vi "UHR-Fleezers Control (host) - Lorentz v2.vi"() -> ()   [LabVIEW 2014] (continued)
                n3918 = String Subset(string=w6021, length (rest)=w6018) -> (substring=w6017:string)  [unwired: 1 out]
                n3919 = Concatenate Strings(w6017, "_log.txt" ("string")) -> (w6015:string)
                n3920 = String To Path(string=w6015) -> (path=w6011:path)
                n3921 = Open/Create/Replace File(file path (use dialog)=w6011, operation (0:open)=T40."create", access (0:read/write)=enum16{"read/write", "read-only", "write-only"}."write-only") -> (refnum out=w6012:refnum<file>)  [unwired: 1 in, 4 out]
                n3922 = Deny Access(7:w6012) -> (3:w6009:refnum<file>)  [unwired: 1 in, 2 out]
                n3923 = call "write to event log.vi"("log file ref"=w6009, "time"=0.0, "input string"="start log") -> ()  [unwired: 8 in]
              }
            }
            "log file ref" <- w5943
            n3924 = Array Size(array=w5979) -> (size(s)=w5980:i32)
            n3925 = Open/Create/Replace File(file path (use dialog)=w5945, operation (0:open)=T40."create", access (0:read/write)=enum16{"read/write", "read-only", "write-only"}."write-only") -> (refnum out=w5993:refnum<file>)  [unwired: 1 in, 4 out]
            n3926 = local write "Saving..."(TRUE ("Saving...")) -> ()
            n3927 = To Double Precision Float(number=w5980) -> (double precision float=w5978:dbl)
            n3928 = String Length(string="Comment (data description)") -> (length=w5977:i32)
            n3929 = To Double Precision Float(number=w5977) -> (double precision float=w5976:dbl)
            n3930 = Deny Access(7:w5993) -> (3:w5992:refnum<file>)  [unwired: 1 in, 2 out]
            n3931 = Build Array (concatenate)(w5978, w5979, w5976) -> (w5955:dbl[])
            n3932 = case "If fluorescence data to be saved" shown="True" w5968 {
              tunnel: w5945 -> [_ w6074]
              tunnel: [w6044 w6057] -> w5969
              tunnel: [w6044 w6045] -> w5941
              frame False {
                w6044 = refnum<k0> refnum
              }
              frame True {
                w6056 = 0.0
                w6049 = T40."create" ("operation (0:open)")
                w6050 = enum16{"read/write", "read-only", "write-only"}."write-only" ("access (0:read/write)")
                n3933 = local read "APD Integration Time (s)"() -> (w6062:dbl)
                n3934 = local read "N APD Samp/step"() -> (w6055:dbl)
                n3935 = local read "Number of APDs"() -> (w6054:u8)
                n3936 = Path To String(path=w6074) -> (string=w6073:string)
                n3937 = String Length(string=w6073) -> (length=w6072:i32)
                n3938 = Subtract(x=w6072, y=4) -> (x-y=w6070:i32)
                n3939 = String Subset(string=w6073, length (rest)=w6070) -> (substring=w6053:string)  [unwired: 1 out]
                n3940 = Build Array(w6062, w6055, w6054, w6056, w6056, w6056, w6056, w6056) -> (w6059:dbl[])
                n3941 = Concatenate Strings(w6053, "_green.dat") -> (w6051:string)
                n3942 = Concatenate Strings(w6053, "_fl.dat" ("string")) -> (w6068:string)
                n3943 = Array Size(array=w6059) -> (size(s)=w6061:i32)
                n3944 = String To Path(string=w6068) -> (path=w6066:path)
                n3945 = Open/Create/Replace File(file path (use dialog)=w6066, operation (0:open)=w6049, access (0:read/write)=w6050) -> (refnum out=w6067:refnum<file>)  [unwired: 1 in, 4 out]
                n3946 = Deny Access(7:w6067) -> (3:w6063:refnum<file>)  [unwired: 1 in, 2 out]
                n3947 = String To Path(string=w6051) -> (path=w6048:path)
                n3948 = To Double Precision Float(number=w6061) -> (double precision float=w6060:dbl)
                n3949 = Build Array (concatenate)(w6060, w6059) -> (w6058:dbl[])
                n3950 = Write to Binary File(file (use dialog)=w6063, data=w6058, 5:FALSE ("prepend array or string size? (T)"), 9:T41."big-endian, network order" ("byte order (0:big-endian, network order)")) -> (refnum out=w6057:refnum<file>)  [unwired: 1 in, 3 out]
                n3951 = Open/Create/Replace File(file path (use dialog)=w6048, operation (0:open)=w6049, access (0:read/write)=w6050) -> (refnum out=w6046:refnum<file>, error out=w6047:errorcluster)  [unwired: 3 in, 1 out]
                n3952 = Deny Access(4:w6047, 7:w6046) -> (3:w6045:refnum<file>)  [unwired: 1 in, 1 out]
              }
            }
            n3953 = case shown="True" w5957 {
              tunnel: w5945 -> [_ w6029]
              tunnel: [refnum<k0> refnum w6028] -> w5958
              frame False {
              }
              frame True {
                w6024 = 0.0 ("element")
                n3954 = Path To String(path=w6029) -> (string=w6043:string)
                n3955 = Build Array(w6024, w6024, w6024, w6024, w6024, w6024, w6024, w6024) -> (w6025:dbl[])
                n3956 = String Length(string=w6043) -> (length=w6042:i32)
                n3957 = Subtract(x=w6042, y=4) -> (x-y=w6040:i32)
                n3958 = Array Size(array=w6025) -> (size(s)=w6027:i32)
                n3959 = String Subset(string=w6043, length (rest)=w6040) -> (substring=w6039:string)  [unwired: 1 out]
                n3960 = To Double Precision Float(number=w6027) -> (double precision float=w6026:dbl)
                n3961 = Concatenate Strings(w6039, "_pos.dat" ("string")) -> (w6037:string)
                n3962 = Build Array (concatenate)(w6026, w6025) -> (w6023:dbl[])
                n3963 = String To Path(string=w6037) -> (path=w6033:path)
                n3964 = Open/Create/Replace File(file path (use dialog)=w6033, operation (0:open)=T40."create", access (0:read/write)=enum16{"read/write", "read-only", "write-only"}."write-only") -> (refnum out=w6034:refnum<file>)  [unwired: 1 in, 4 out]
                n3965 = Deny Access(7:w6034) -> (3:w6030:refnum<file>)  [unwired: 1 in, 2 out]
                n3966 = Write to Binary File(file (use dialog)=w6030, data=w6023, 5:FALSE ("prepend array or string size? (T)"), 9:T41."big-endian, network order" ("byte order (0:big-endian, network order)")) -> (refnum out=w6028:refnum<file>)  [unwired: 1 in, 3 out]
              }
            }
            n3967 = Write to Binary File(file (use dialog)=w5992, data=w5955, 5:w5974, 9:w5973) -> (refnum out=w5975:refnum<file>)  [unwired: 1 in, 3 out]
            n3968 = Write to Binary File(file (use dialog)=w5975, data="Comment (data description)", 5:w5974, 9:w5973) -> (refnum out=w5972:refnum<file>)  [unwired: 1 in, 3 out]
            n3969 = local read "connection reference"() -> (w5956:T21)
            n3970 = Bundle("Comment (data description)"="Comment (data description)", "Channel 1 Buffer"="Channel 1 Buffer", "Channel 2 Buffer"="Channel 2 Buffer", "Channel 3 Buffer"="Channel 3 Buffer", "Title"="Title", "DNA Construct"="DNA Construct", "Bead diameter"="Bead diameter", "Name"="Name") -> (w5946:T63)  [unwired: 1 in]
            n3971 = disable-structure shown="Disabled" {
              disable-tunnel: w5956 -> [w6004 _]
              disable-tunnel: w5955 -> [w6002 _]
              disable-tunnel: w5946 -> [w6001 _]
              disable-tunnel: w5945 -> [w6000 _]
              frame Disabled {
                n3972 = call "MattFileCreator-v9.vi"("Comments"=w6001, "Input Array"=w6002, "File path"=w6000, "table"="labview", "connection reference"=w6004) -> ("connection reference out"=w6003:T21)  [unwired: 5 in, 1 out]
                n3973 = local write "connection reference"(w6003) -> ()
              }
              frame Enabled {
              }
            }
          }
        }
        n3974 = feedback-in #29(w5898) -> ()
        n3975 = feedback-in #30(w5924) -> ()
        n3976 = feedback-in #31(w5907) -> ()
        n3977 = feedback-in #32(w5923) -> ()
        n3978 = feedback-in #33(w5913) -> ()
        n3979 = feedback-in #34(w5891) -> ()
        n3980 = feedback-in #35(w5897) -> ()
        n3981 = feedback-in #36(w5887) -> ()
        n3982 = feedback-in #37(w5910) -> ()
      }
      frame #1 {
        n3983 = local read "Saving..."() -> (w6233:bool)
        n3984 = case shown="True" w6233 {
          tunnel: w6237 -> [_ w6252]
          tunnel: w6236 -> [_ w6266]
          tunnel: w6235 -> [_ w6262]
          tunnel: w6234 -> [_ w6261]
          tunnel: w6232 -> [_ w6260]
          tunnel: w6231 -> [_ w6255]
          tunnel: w6230 -> [_ w6254]
          tunnel: w6229 -> [_ w6253]
          tunnel: w6228 -> [_ w6251]
          tunnel: w6227 -> [_ w6249]
          tunnel: w6226 -> [_ w6248]
          tunnel: w6225 -> [_ w6247]
          tunnel: w6224 -> [_ w6246]
          tunnel: w6223 -> [_ w6245]
          tunnel: w6222 -> [_ w6244]
          tunnel: w6221 -> [_ w6243]
          tunnel: w6220 -> [_ w6242]
          tunnel: w6219 -> [_ w6240]
          tunnel: w6218 -> [_ w6239]
          tunnel: w6217 -> [_ w6238]
          frame False {
          }
          frame True {
            n3985 = case shown="True" "Stop saving data + video" {
              frame False {
              }
              frame True {
                n3986 = local write "Save Video"(FALSE ("Save Video")) -> ()
              }
            }
            n3987 = Multiply(x=w6252, y=w6251) -> (x*y=→"Time (s)":dbl)
            n3988 = Less Or Equal?(x=w6252, y=w6260) -> (x <= y?=w6264:bool)
            n3989 = Compound Arithmetic op=OR("Stop Saving", "Abort save 2", "Stop saving data + video") -> (w6256:bool)
            n3990 = Not(x=w6256) -> (.not. x?=w6265:bool)
            n3991 = And(x=w6264, y=w6265) -> (x .and. y?=w6263:bool)
            n3992 = case shown="True" w6263 {
              tunnel: w6266 -> [w6277 w6378]
              tunnel: [0.0 w6381] -> w6259
              tunnel: w6252 -> [_ w6379]
              tunnel: w6260 -> [_ w6380]
              tunnel: w6262 -> [_ w6375]
              tunnel: w6261 -> [_ _]
              tunnel: w6255 -> [w6275 w6368]
              tunnel: w6254 -> [w6274 w6369]
              tunnel: w6253 -> [_ w6367]
              tunnel: w6249 -> [_ w6366]
              tunnel: w6248 -> [_ w6284]
              tunnel: w6247 -> [_ w6359]
              tunnel: w6246 -> [_ w6306]
              tunnel: w6245 -> [w6271 w6323]
              tunnel: w6244 -> [w6272 w6322]
              tunnel: w6243 -> [_ w6319]
              tunnel: w6242 -> [_ w6317]
              tunnel: w6240 -> [_ w6283]
              tunnel: w6239 -> [w6270 _]
              tunnel: w6238 -> [w6268 w6282]
              frame False {
                w6273 = FALSE
                n3993 = Close File(refnum=w6277) -> ()  [unwired: 1 in, 2 out]
                n3994 = case shown="True" w6274 {
                  tunnel: w6275 -> [_ w6281]
                  tunnel: w6268 -> [_ w6280]
                  frame False {
                  }
                  frame True {
                    n3995 = Close File(refnum=w6281) -> ()  [unwired: 1 in, 2 out]
                    n3996 = Close File(refnum=w6280) -> ()  [unwired: 1 in, 2 out]
                  }
                }
                n3997 = case shown="True" w6271 {
                  tunnel: w6272 -> [_ w6279]
                  frame False {
                  }
                  frame True {
                    n3998 = Close File(refnum=w6279) -> ()  [unwired: 1 in, 2 out]
                  }
                }
                n3999 = local read "Save Event Log?"() -> (w6269:bool)
                n4000 = case shown="True" w6269 {
                  tunnel: w6270 -> [_ w6278]
                  frame False {
                  }
                  frame True {
                    n4001 = Close File(refnum=w6278) -> ()  [unwired: 1 in, 2 out]
                  }
                }
                n4002 = local write "Raster Scanning..."(w6273) -> ()
                n4003 = local write "Calibrating Trap..."(w6273) -> ()
                n4004 = call <vilib>:"Beep.vi"() -> ()  [unwired: 3 in, 9 out]
                n4005 = local write "Stop Saving"(w6273) -> ()
                "Saving..." <- w6273
              }
              frame True {
                n4006 = local read "Calibrating Trap..."() -> (w6370:bool)
                n4007 = case "Write fl. data" shown="True" w6369 {
                  tunnel: w6368 -> [_ w6411]
                  tunnel: w6367 -> [_ w6410]
                  tunnel: w6282 -> [_ w6404]
                  frame False {
                  }
                  frame True {
                    w6403 = FALSE ("prepend array or string size? (T)")
                    w6405 = T41."big-endian, network order" ("byte order (0:big-endian, network order)")
                    n4008 = property on="Green Laser ON" class="Bool (strict)"() -> ("Value"=w6409:bool)  [unwired: 2 in, 2 out]
                    n4009 = property on="Green Intensity % (FB OFF)" class="DigNum (strict)"() -> ("Value"=w6408:dbl)  [unwired: 2 in, 2 out]
                    n4010 = Boolean To (0,1)(Boolean=w6409) -> (0, 1=w6407:i16)
                    n4011 = Multiply(x=w6407, y=w6408) -> (x*y=w6406:dbl)
                    n4012 = Write to Binary File(file (use dialog)=w6411, data=w6410, 5:w6403, 9:w6405) -> ()  [unwired: 1 in, 4 out]
                    n4013 = Write to Binary File(file (use dialog)=w6404, data=w6406, 5:w6403, 9:w6405) -> ()  [unwired: 2 in, 3 out]
                  }
                }
                n4014 = Greater?(x="Save ave N", y=1.0) -> (0:w6373:bool)
                n4015 = Not(x=w6370) -> (.not. x?=w6372:bool)
                n4016 = And(x=w6372, y=w6373) -> (x .and. y?=w6320:bool)
                n4017 = case shown="True" w6320 {
                  tunnel: w6319 -> [w6384 w6395]
                  tunnel: [w6384 w6387] -> w6318
                  tunnel: "Save ave N" -> [_ w6388]
                  frame False {
                  }
                  frame True {
                    w6385 = 2 ("dimension size")
                    n4018 = Array Size(array=w6395) -> (size(s)=w6389:i32)
                    n4019 = Divide(x=w6389, y=w6385) -> (x/y=w6393:dbl)
                    n4020 = Reshape Array(w6395, w6393, w6385) -> (w6394:u64[][])
                    n4021 = Transpose 2D Array(2D array=w6394) -> (transposed array=w6392:u64[][])
                    n4022 = for {
                      tunnel: w6392 -> [w6397] mode=indexing
                      tunnel: [w6396] -> w6386 mode=indexing
                      tunnel: w6388 -> [w6398]
                      workers-P: _ -> [_]
                      n4023 = call "downsample 1D array - U64.vi"("Ave N"=w6398, "Array In"=w6397) -> ("Array Out"=w6396:u64[])  [unwired: 1 in]
                    }
                    n4024 = Transpose 2D Array(2D array=w6386) -> (transposed array=w6391:u64[][])
                    n4025 = Divide(x=w6389, y=w6388) -> (x/y=w6390:dbl)
                    n4026 = Reshape Array(w6391, w6390) -> (w6387:u64[])
                  }
                }
                n4027 = case shown="True" w6320 {
                  tunnel: w6375 -> [w6412 w6424]
                  tunnel: [w6412 w6416] -> w6371
                  tunnel: "Save ave N" -> [_ w6417]
                  tunnel: w6366 -> [_ w6415]
                  frame False {
                  }
                  frame True {
                    n4028 = Array Size(array=w6424) -> (size(s)=w6418:i32)
                    n4029 = Array Size(array=w6415) -> (size(s)=w6414:i32)
                    n4030 = Divide(x=w6418, y=w6414) -> (x/y=w6422:dbl)
                    n4031 = Reshape Array(w6424, w6422, w6414) -> (w6423:dbl[][])
                    n4032 = Transpose 2D Array(2D array=w6423) -> (transposed array=w6421:dbl[][])
                    n4033 = for {
                      tunnel: w6421 -> [w6427] mode=indexing
                      tunnel: [w6426] -> w6413 mode=indexing
                      tunnel: w6417 -> [w6425]
                      workers-P: _ -> [_]
                      n4034 = call "downsample 1D array - I16 to F32.vi"("Ave N"=w6425, "Array In"=w6427) -> ("Array Out"=w6426:sgl[])  [unwired: 1 in]
                    }
                    n4035 = Transpose 2D Array(2D array=w6413) -> (transposed array=w6420:sgl[][])
                    n4036 = Divide(x=w6418, y=w6417) -> (x/y=w6419:dbl)
                    n4037 = Reshape Array(w6420, w6419) -> (w6416:sgl[])
                  }
                }
                n4038 = Index Array(array=w6306, index=2) -> (element=w6307:waveform(dbl))
                n4039 = Index Array(array=w6306, index=1) -> (element=w6340:waveform(dbl))
                n4040 = Index Array(array=w6306, index=0) -> (element=w6342:waveform(dbl))
                n4041 = Unbundle By Name(w6307) -> ("Y"=w6309:dbl[])
                n4042 = Unbundle By Name(w6340) -> ("Y"=w6344:dbl[])
                n4043 = Unbundle By Name(w6342) -> ("Y"=w6352:dbl[])
                n4044 = case "Write trap pos. data" shown="True" w6323 {
                  tunnel: w6322 -> [_ w6400]
                  tunnel: w6318 -> [_ w6399]
                  frame False {
                  }
                  frame True {
                    n4045 = Write to Binary File(file (use dialog)=w6400, data=w6399, 5:FALSE ("prepend array or string size? (T)"), 9:T41."big-endian, network order" ("byte order (0:big-endian, network order)")) -> ()  [unwired: 1 in, 4 out]
                  }
                }
                n4046 = Write to Binary File(file (use dialog)=w6378, data=w6371, 5:FALSE ("prepend array or string size? (T)"), 9:T41."big-endian, network order" ("byte order (0:big-endian, network order)")) -> ()  [unwired: 1 in, 4 out]
                n4047 = feedback #38(w6309) -> (w6310:dbl[])
                n4048 = Build Array (concatenate)(w6310, w6309) -> (w6305:dbl[])
                n4049 = Select(t=w6309, s=w6284, f=w6305) -> (s? t:f=w6295:dbl[])
                n4050 = feedback-in #38(w6295) -> ()
                n4051 = feedback #39(w6344) -> (w6346:dbl[])
                n4052 = Build Array (concatenate)(w6346, w6344) -> (w6345:dbl[])
                n4053 = Select(t=w6344, s=w6284, f=w6345) -> (s? t:f=w6334:dbl[])
                n4054 = feedback-in #39(w6334) -> ()
                n4055 = feedback #40(w6352) -> (w6365:dbl[])
                n4056 = Build Array (concatenate)(w6365, w6352) -> (w6364:dbl[])
                n4057 = Select(t=w6352, s=w6284, f=w6364) -> (s? t:f=w6339:dbl[])
                n4058 = feedback-in #40(w6339) -> ()
                n4059 = Divide(x=w6379, y=w6380) -> (x/y=w6382:dbl)
                n4060 = Multiply(x=w6382, y=100.0) -> (x*y=w6381:dbl)
                n4061 = Build Array(w6339, w6334, w6295) -> (→"Saved APD":dbl[][])
                n4062 = Array Size(array=w6339) -> (size(s)=w6357:i32)
                n4063 = Unbundle By Name(w6359) -> ("Y"=w6363:dbl[])
                n4064 = Subtract(x=w6357, y="N pts to average") -> (x-y=w6292:i32)
                n4065 = Multiply(x="N pts to average", y=u16 2) -> (x*y=w6335:u16)
                n4066 = Subtract(x=w6357, y=w6335) -> (x-y=w6293:i32)
                n4067 = feedback #41(w6363) -> (w6362:dbl[])
                n4068 = Build Array (concatenate)(w6362, w6363) -> (w6361:dbl[])
                n4069 = Select(t=w6363, s=w6284, f=w6361) -> (s? t:f=w6360:dbl[])
                "Trap Delta Graph" <- w6360
                n4070 = feedback-in #41(w6360) -> ()
                n4071 = Array Subset(array=w6339, index=w6292, length="N pts to average") -> (w6356:dbl[])
                n4072 = Array Subset(array=w6339, index=w6293, length="N pts to average") -> (w6355:dbl[])
                n4073 = Array Subset(array=w6334, index=w6292, length="N pts to average") -> (w6337:dbl[])
                n4074 = Array Subset(array=w6334, index=w6293, length="N pts to average") -> (w6336:dbl[])
                n4075 = Array Subset(array=w6295, index=w6292, length="N pts to average") -> (w6304:dbl[])
                n4076 = Array Subset(array=w6295, index=w6293, length="N pts to average") -> (w6303:dbl[])
                n4077 = Index Array(array=w6317, index=0) -> (element=w6315:waveform(dbl))
                n4078 = call-poly <vilib>:"Mean.vi"("X"=w6356) -> ("mean"=w6354:dbl)  [unwired: 1 out]
                n4079 = call-poly <vilib>:"Mean.vi"("X"=w6337) -> ("mean"=w6333:dbl)  [unwired: 1 out]
                n4080 = call-poly <vilib>:"Mean.vi"("X"=w6355) -> ("mean"=w6353:dbl)  [unwired: 1 out]
                n4081 = call-poly <vilib>:"Mean.vi"("X"=w6336) -> ("mean"=w6332:dbl)  [unwired: 1 out]
                n4082 = call-poly <vilib>:"Mean.vi"("X"=w6304) -> ("mean"=w6302:dbl)  [unwired: 1 out]
                n4083 = call-poly <vilib>:"Mean.vi"("X"=w6303) -> ("mean"=w6301:dbl)  [unwired: 1 out]
                n4084 = Unbundle By Name(w6315) -> ("Y"=w6313:dbl[])
                n4085 = Subtract(x=w6333, y=w6332) -> (x-y=w6324:dbl)
                "Delta Fl. 2" <- w6324
                n4086 = Subtract(x=w6302, y=w6301) -> (x-y=w6296:dbl)
                "Delta Fl. 3" <- w6296
                n4087 = Subtract(x=w6354, y=w6353) -> (x-y=w6351:dbl)
                "Delta Fl. 1" <- w6351
                n4088 = feedback #42(w6313) -> (w6312:dbl[])
                n4089 = Build Array (concatenate)(w6312, w6313) -> (w6314:dbl[])
                n4090 = Initialize Array(w6351, 1 ("dimension size")) -> (w6348:dbl[])
                n4091 = Initialize Array(w6324, 1 ("dimension size")) -> (w6329:dbl[])
                n4092 = Initialize Array(w6296, 1 ("dimension size")) -> (w6298:dbl[])
                n4093 = Select(t=w6313, s=w6284, f=w6314) -> (s? t:f=w6311:dbl[])
                "Saved trap pos" <- w6311
                n4094 = feedback-in #42(w6311) -> ()
                n4095 = feedback #43(w6348) -> (w6349:dbl[])
                n4096 = Build Array (concatenate)(w6349, w6348) -> (w6347:dbl[])
                n4097 = feedback #44(w6329) -> (w6330:dbl[])
                n4098 = feedback #45(w6298) -> (w6299:dbl[])
                n4099 = Build Array (concatenate)(w6330, w6329) -> (w6328:dbl[])
                n4100 = Build Array (concatenate)(w6299, w6298) -> (w6297:dbl[])
                n4101 = Select(t=w6348, s=w6284, f=w6347) -> (s? t:f=w6327:dbl[])
                n4102 = feedback-in #43(w6327) -> ()
                n4103 = Select(t=w6329, s=w6284, f=w6328) -> (s? t:f=w6326:dbl[])
                n4104 = feedback-in #44(w6326) -> ()
                n4105 = Select(t=w6298, s=w6284, f=w6297) -> (s? t:f=w6291:dbl[])
                n4106 = feedback-in #45(w6291) -> ()
                n4107 = Build Array(w6327, w6326, w6291) -> (→"Save APD Deriv":dbl[][])
                n4108 = Index Array(array=w6283, index=15) -> (element=w6289:waveform(dbl))
                n4109 = Unbundle By Name(w6289) -> ("Y"=w6287:dbl[])
                n4110 = feedback #46(w6287) -> (w6286:dbl[])
                n4111 = Build Array (concatenate)(w6286, w6287) -> (w6288:dbl[])
                n4112 = Select(t=w6287, s=w6284, f=w6288) -> (s? t:f=w6285:dbl[])
                "Amp current" <- w6285
                n4113 = feedback-in #46(w6285) -> ()
              }
            }
            "Progress" <- w6259
            "Progress 2" <- w6259
          }
        }
      }
    }
    n4114 = local read "wait to reset values"() -> (w4761:bool)
    n4115 = Not(x=w4759) -> (.not. x?=w4762:bool)
    n4116 = And(x=w4762, y=w4761) -> (x .and. y?=w4763:bool)
    n4117 = case "Part of MCL raster scanning: returns to initial positions after scan done" shown="True" w4763 {
      tunnel: w4390 -> [w5708 w5715]
      tunnel: [w5708 w5714] -> w4765
      tunnel: w4532 -> [w5707 w5713]
      tunnel: [w5707 w5712] -> w4760
      frame False {
      }
      frame True {
        w5723 = 10.0 ("y")
        w5722 = 32767.0 ("y")
        # "to return scan values\nafter a synchronous \nAOM scan"
        n4118 = local read "AO2"() -> (w5716:dbl)
        n4119 = local read "AO1"() -> (w5717:dbl)
        n4120 = local write "wait to reset values"(FALSE ("wait to reset values")) -> ()
        n4121 = Multiply(x=w5717, y=w5722) -> (x*y=w5719:dbl)
        n4122 = Multiply(x=w5716, y=w5722) -> (x*y=w5721:dbl)
        n4123 = Divide(x=w5719, y=w5723) -> (x/y=w5718:dbl)
        n4124 = Divide(x=w5721, y=w5723) -> (x/y=w5720:dbl)
        n4125 = To Word Integer(number=w5718) -> (16bit integer=w5724:i16)
        n4126 = To Word Integer(number=w5720) -> (16bit integer=w5725:i16)
        n4127 = local read "Total Counts (ticks)"() -> (w5709:u16)
        n4128 = local read "Scan Range (V)\n(of steps)"() -> (w5710:dbl)
        n4129 = xnode "Read/Write Control"("FPGA VI Reference In"=w5715, "error in"=w5713, "AO1"=w5724, "AO2"=w5725, "MCL count"=w5709) -> ("FPGA VI Reference Out"=w5714:T31, "error out"=w5712:errorcluster)
        n4130 = property on="Scan Range (V)\n(of steps)" class="DigNum (strict)"("Val(Sgnl)"=w5710) -> ()  [unwired: 2 in, 2 out]
      }
    }
    n4131 = case shown="True" "Sound ON" {
      tunnel: [w4836 w4881] -> w4459
      tunnel: w4458 -> [w4836 w4880]
      tunnel: w4456 -> [_ _]
      tunnel: w4434 -> [_ w4839]
      tunnel: w4455 -> [_ _]
      tunnel: w4454 -> [_ w4850]
      tunnel: w4453 -> [_ w4860]
      frame False {
      }
      frame True {
        n4132 = Index Array(array=w4839, index="Data channel to sound") -> (element=w4838:waveform(dbl))
        "Waveform Graph 2" <- w4838
        n4133 = Unbundle By Name(w4838) -> ("dt"=w4864:dbl, "Y"=w4862:dbl[])
        n4134 = Array Size(array=w4862) -> (size(s)=w4863:i32)
        "N data samples" <- w4863
        n4135 = for "Data time base" {
          N: w4863 -> [_]
          tunnel: [w4885] -> w4865 mode=indexing
          i -> [w4885]
        }
        n4136 = Multiply(x=w4864, y=w4865) -> (x*y=w4861:dbl[])
        n4137 = Compound Arithmetic op=MULTIPLY(6.283185307179586, "Carrier Frequency (Hz)", w4860) -> (w4877:dbl[])
        n4138 = call <vilib>:"Interpolate 1D.vi"("X is monotonic"=TRUE, "xi"=w4860, "X"=w4861, "Y"=w4862) -> ("yi"=w4858:dbl[])  [unwired: 5 in, 2 out]
        n4139 = Sine(x=w4877) -> (sin(x)=w4866:dbl[])
        n4140 = Add(x=w4858, y="Offset") -> (x+y=w4856:dbl[])
        n4141 = Multiply(x=w4856, y="mult x") -> (x*y=w4854:dbl[])
        n4142 = Add(x="Offset 2", y=w4854) -> (x+y=w4849:dbl[])
        n4143 = Compound Arithmetic op=MULTIPLY(6.283185307179586, "Carrier Frequency (Hz)", w4850, w4849) -> (w4841:dbl[])
        n4144 = for "Cumulative sum" {
          tunnel: [w4884] -> w4847 mode=indexing
          shift-right: [w4884] -> w4844
          shift-left: 0.0 -> [w4883]
          tunnel: w4841 -> [w4882] mode=indexing
          n4145 = Add(x=w4882, y=w4883) -> (x+y=w4884:dbl)
        }
        n4146 = feedback #47(0.0) -> (w4843:dbl)
        n4147 = Add(x=w4847, y=w4843) -> (x+y=w4846:dbl[])
        n4148 = Add(x=w4844, y=w4843) -> (x+y=w4842:dbl)
        n4149 = feedback-in #47(w4842) -> ()
        n4150 = Sine(x=w4846) -> (sin(x)=w4840:dbl[])
        n4151 = Select(t=w4866, s="tone or data", f=w4840) -> (s? t:f=w4872:dbl[])
        n4152 = Multiply(x=w4872, y="Volume") -> (x*y=w4870:dbl[])
        n4153 = Initialize Array(0.0 ("element"), "N initial buffer elements") -> (w4873:dbl[])
        n4154 = Multiply(x="N initial buffer elements", y=w4850) -> (x*y=→"Initial buffer time (s)":dbl)
        n4155 = Build Array (concatenate)(w4873, w4870) -> (w4875:dbl[])
        n4156 = First Call?() -> (First Call?: T/F=w4876:bool)
        n4157 = Select(t=w4875, s=w4876, f=w4870) -> (s? t:f=w4869:dbl[])
        n4158 = call-poly <vilib>:"Sound Output Write.vi"("data"=w4869, "task ID"=w4880) -> ("task ID out"=w4881:T50)  [unwired: 8 in, 1 out]
      }
    }
    n4159 = node-c288() -> ()  [unwired: 2 out]
  }
  n4160 = disable-structure shown="Disabled" {
    disable-tunnel: w16 -> [w6428 _]
    frame Disabled {
      n4161 = call <vilib>:"Sound Output Clear.vi"("task ID"=w6428) -> ()  [unwired: 10 in, 1 out]
    }
    frame Enabled {
    }
  }
  n4162 = node-c288(w59) -> ()  [unwired: 1 out]
  n4163 = node-c288(w67) -> ()  [unwired: 1 out]
  n4164 = flat-sequence {
    tunnel: w74 -> [w6432]
    tunnel: w75 -> [w6433]
    tunnel: [w6431] -> w73
    tunnel: [w6430] -> w72
    tunnel: w71 -> [_]
    tunnel: w69 -> [_]
    tunnel: w65 -> [_]
    tunnel: w73 -> [w6434]
    tunnel: w72 -> [w6435]
    frame #0 {
      w6429 = FALSE ("AI to FIFO")
      n4165 = xnode "Read/Write Control"("FPGA VI Reference In"=w6433, "error in"=w6432, "AI to FIFO"=w6429, "APD to FIFO"=w6429) -> ("FPGA VI Reference Out"=w6431:T31, "error out"=w6430:errorcluster)
    }
    frame #1 {
      n4166 = xnode "Close FPGA VI Reference"("FPGA VI Reference In"=w6434, "error in"=w6435) -> ("error out"=→"error out":errorcluster)
    }
  }
